vi "Convert to C code.vi"(8 "Error In":errorcluster) -> (0 "Error Out":errorcluster)   [LabVIEW 2014, in "ESP8266 WiFi Wrapper.lvlib"]
uses:
  ESP8266 WiFi Wrapper.lvlib
panel:
  out "transcripted code":string
  in  "Defines":string[](array[string])=["using namespace std;"]
  in  "Includes":string[](array[string])=["<ArduinoSTL.h>", "<vector.h>"]
  in  "vi path":path
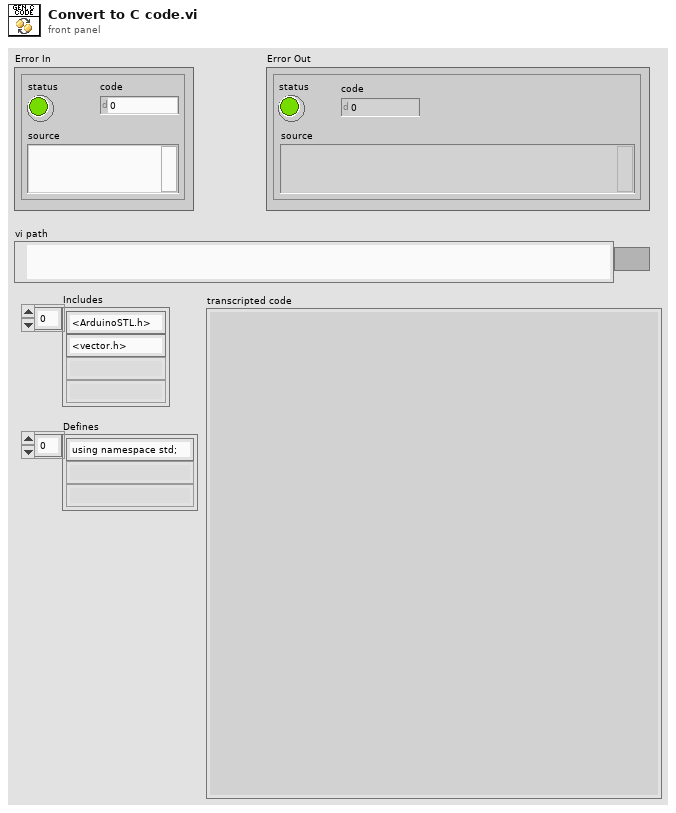
[diagram p1: front panel]
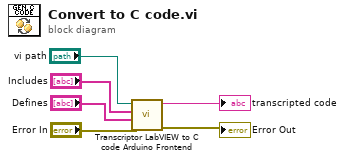
[diagram p0: block diagram]
diagram:
  n1 = call <vilib>:"Transcriptor LabVIEW to C code Arduino Frontend.vi"("error in"="Error In", "Defines"="Defines", "Includes"="Includes", "vi path"="vi path") -> ("error out"=→"Error Out":errorcluster, "transcripted code"=→"transcripted code":string)  [unwired: 6 in]
